vi "detrend.vi"(11 "Array in":sgl[](array[numeric])) -> (3 "Array out":sgl[](array[numeric]))   [LabVIEW 2013]
uses:
  <vilib>/Analysis/NI_AALPro.lvlib
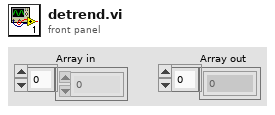
[diagram p1: front panel]
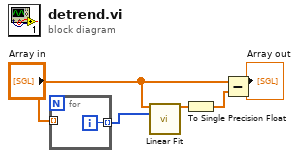
[diagram p0: block diagram]
diagram:
  n1 = for {
    tunnel: "Array in" -> [_] mode=indexing
    tunnel: [w6] -> w1 mode=indexing
    i -> [w6]
  }
  n2 = call <vilib>:"Linear Fit.vi"("Y"="Array in", "X"=w1) -> ("Best Linear Fit"=w5:dbl[])  [unwired: 9 in, 4 out]
  n3 = To Single Precision Float(number=w5) -> (single precision float=w4:sgl[])
  n4 = Subtract(x="Array in", y=w4) -> (x-y=→"Array out":sgl[])
